vi "Read Code.vi"(8 "error in (no error)":errorcluster, 11 "baseParser in":refnum<class "baseParser.lvclass">) -> (0 "error out":errorcluster, 2 "Code":string, 3 "baseParser out":refnum<class "baseParser.lvclass">)   [LabVIEW 2013, in "baseParser.lvclass"]
uses:
  baseParser.lvclass
  baseParser.lvclass/baseParser.ctl
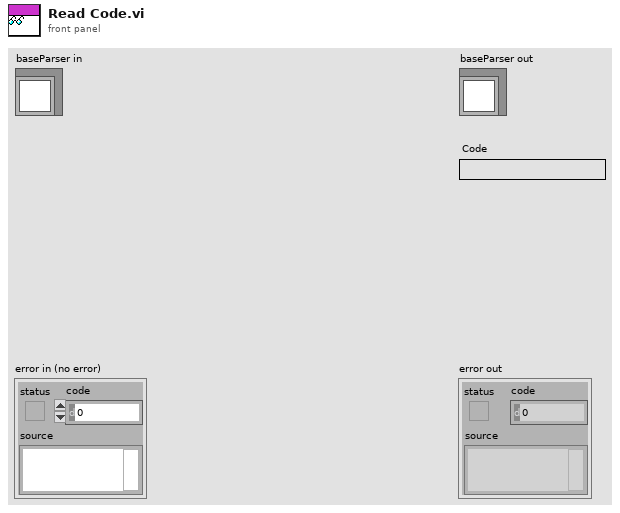
[diagram p1: front panel]
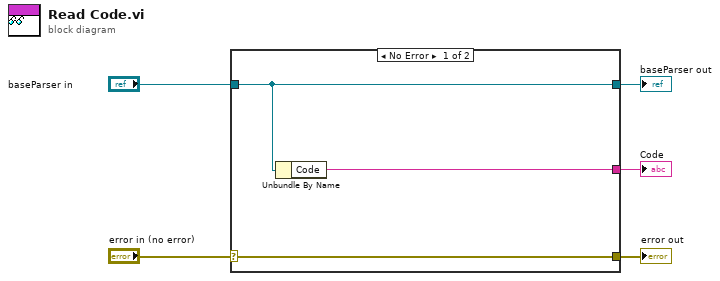
[diagram p0: block diagram]
diagram:
  n1 = case shown="No Error" "error in (no error)" {
    selector: "error in (no error)" -> [w8 w9]
    tunnel: [w8 w9] -> w4
    tunnel: [w7 w10] -> w2
    tunnel: "baseParser in" -> [w7 w10]
    tunnel: [w6 _] -> w1
    frame No Error {
      n2 = Unbundle By Name(w7) -> ("Code"=w6:string)
    }
    frame Error {
    }
  }
  "error out" <- w4
  "baseParser out" <- w2
  "Code" <- w1
